vi "test_dll.vi"() -> ()   [LabVIEW 2018]
panel:
  in  "Slide 3":dbl(slide) scale=0.0..10.0
  out "python return value":dbl(knob) scale=0.0..4000.0
  out "python node FPS":dbl(knob) scale=1.0..10000000.0 scale format="%#_6f"
  in  "python node stop":bool
  out "dll node FPS":dbl(knob) scale=1.0..10000000.0 scale format="%#_6f"
  in  "dll node stop":bool
  in  "dll vi in1":dbl(slide) scale=0.0..10.0
  out "dll vi return value":dbl(knob) scale=0.0..4000.0
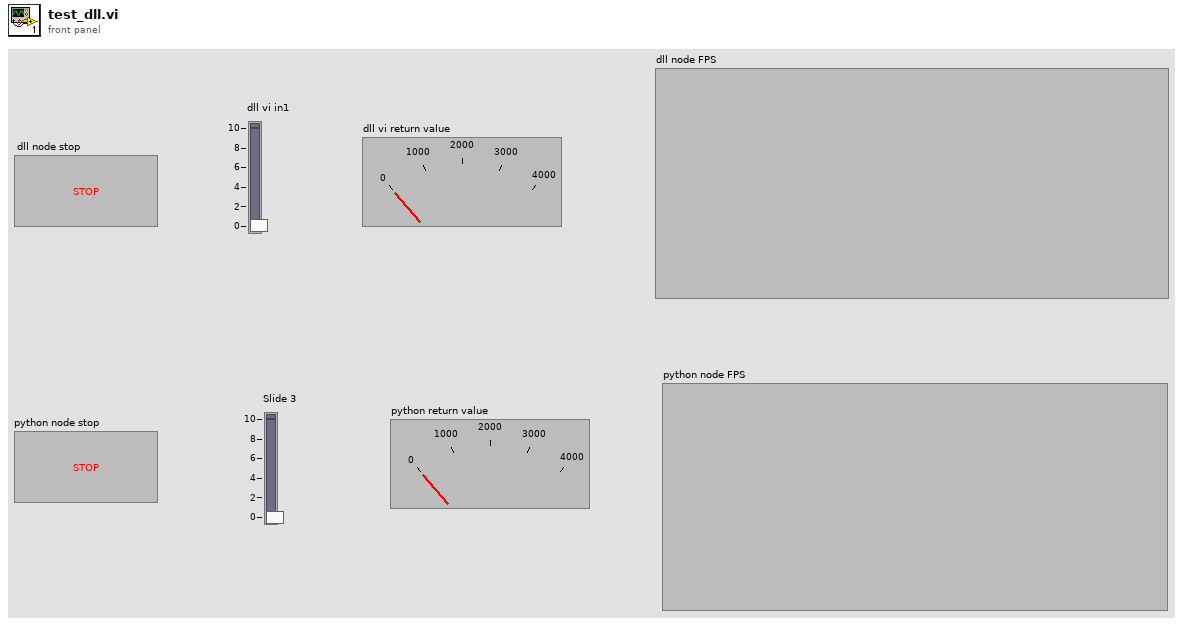
[diagram p1: front panel]
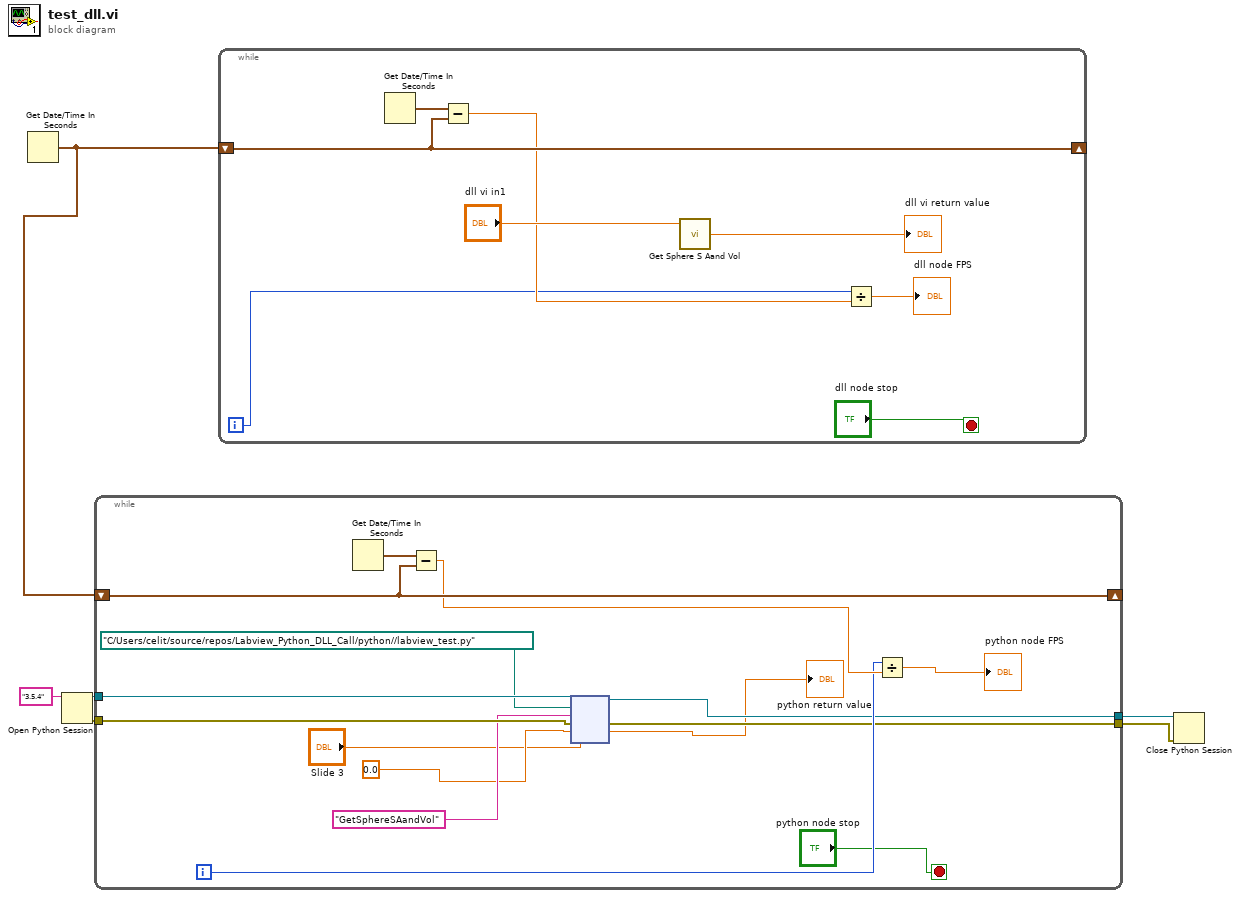
[diagram p0: block diagram]
diagram:
  n1 = Get Date/Time In Seconds() -> (seconds since 1Jan1904=w1:timestamp)
  n2 = Open Python Session(python version="3.5.4" ("Python version")) -> (session out=w5:refnum<k35>, error out=w3:errorcluster)  [unwired: 2 in]
  n3 = while {
    shift-right: [w20] -> _
    shift-left: w1 -> [w20]
    tunnel: w5 -> [w15]
    tunnel: [w14] -> w4
    tunnel: w3 -> [w13]
    tunnel: [w12] -> w2
    i -> [w18]
    stop <- "python node stop" stop-if-true
    n4 = Get Date/Time In Seconds() -> (seconds since 1Jan1904=w21:timestamp)
    n5 = Subtract(x=w21, y=w20) -> (x-y=w19:dbl)
    n6 = node ("Python Node")(w15, path "C:/Users/celit/source/repos/Labview_Python_DLL_Call/python//labview_test.py" ("module path"), "GetSphereSAandVol" ("function name"), w13, 0.0, "Slide 3") -> (w14:refnum<k35>, w12:errorcluster, →"python return value":dbl)  [unwired: 1 in, 2 out]
    n7 = Divide(x=w18, y=w19) -> (x/y=→"python node FPS":dbl)
  }
  n8 = while {
    shift-right: [w26] -> _
    shift-left: w1 -> [w26]
    i -> [w24]
    stop <- "dll node stop" stop-if-true
    n9 = Get Date/Time In Seconds() -> (seconds since 1Jan1904=w27:timestamp)
    n10 = Subtract(x=w27, y=w26) -> (x-y=w25:dbl)
    n11 = call "Get Sphere S Aand Vol.vi"("radius"="dll vi in1") -> ("vol out"=→"dll vi return value":dbl)  [unwired: 2 in, 2 out]
    n12 = Divide(x=w24, y=w25) -> (x/y=→"dll node FPS":dbl)
  }
  n13 = Close Python Session(session in=w4, error in=w2) -> ()  [unwired: 1 out]
